vi "Analog DAQ_Read.vi"(0 "Analog DAQ In":refnum<class "FTW-ActorConnector.lvclass">, 11 "error in (no error)":errorcluster) -> (4 "Analog DAQ Out":refnum<class "FTW-ActorConnector.lvclass">, 8 "Current Value":dbl format="%0.2f", 15 "error out":errorcluster)   [LabVIEW 2018]
uses:
  source/actor/Connector/FTW-ActorConnector.lvclass
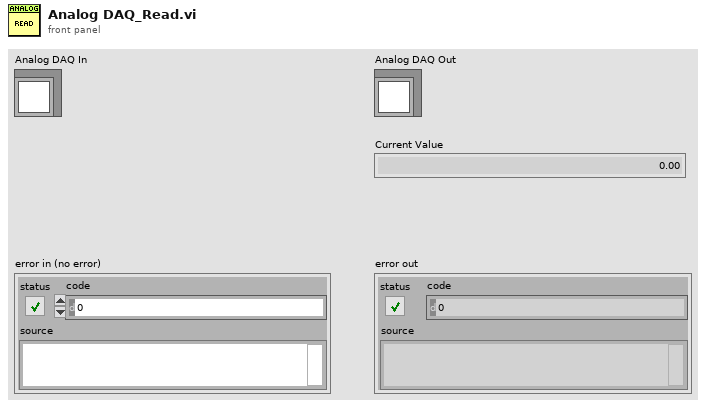
[diagram p1: front panel]
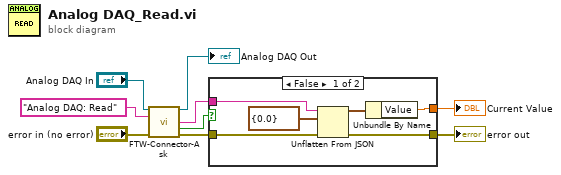
[diagram p0: block diagram]
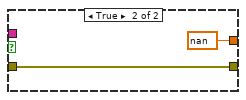
[diagram p2: hidden frame]
diagram:
  n1 = call "FTW-Connector-Ask.vi"("FTW Actor Connector"="Analog DAQ In", "Request Header"="Analog DAQ: Read", "error in"="error in (no error)") -> ("FTW Actor Connector out"=→"Analog DAQ Out":refnum<class "FTW-ActorConnector.lvclass">, "Response Body"=w2:string, "Timed out?"=w1:bool, "error out"=w4:errorcluster)  [unwired: 7 in, 2 out]
  n2 = case shown="False" w1 {
    tunnel: w4 -> [w15 w17]
    tunnel: [w14 w17] -> w6
    tunnel: w2 -> [w13 _]
    tunnel: [w10 nan ("Value")] -> w5
    frame False {
      n3 = Unflatten From JSON(JSON string=w13, type and defaults=cluster{"Value":dbl} {"Value"=0.0}, error in (no error)=w15) -> (value=w11:cluster{"Value":dbl}, error out=w14:errorcluster)  [unwired: 4 in]
      n4 = Unbundle By Name(w11) -> ("Value"=w10:dbl)
    }
    frame True {
    }
  }
  "error out" <- w6
  "Current Value" <- w5
